vi "REF_EDITOR_prepare_DELETE_transaction.vi"(7 "nmb_of_top_rows (all)":i32, 8 "error_in":errorcluster, 10 "selected_record":i32, 11 "REF_EDIT_records":string[][](array[string])) -> (0 "error_out":errorcluster, 3 "DELETE_transaction":string[](array[string]))   [LabVIEW 2019]
uses:
  FGV/REF_EDITOR_records_display/FGV_REF_EDITOR_records_display.ctl
  FGV/login/FGV_login.ctl
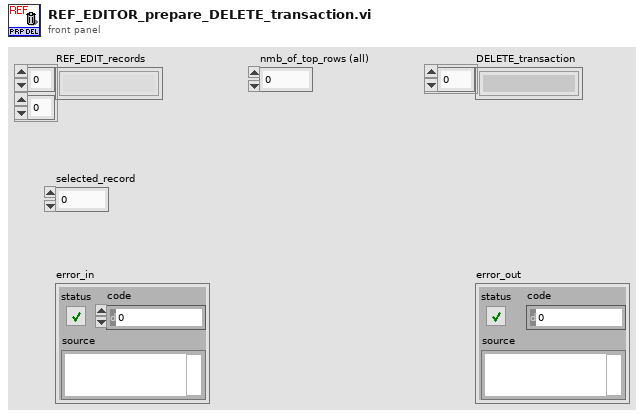
[diagram p1: front panel]
types:
  T1 = typedef "FGV_login.ctl" = enum16{"initialize", "login", "logout", "get_login_info"}
  T2 = typedef "FGV_REF_EDITOR_records_display.ctl" = enum16{"initialize", "set_reference_tables_names", "set_station_number", "set_type_filter", "set_headers", "set_records", "get_ref_table_name", "get_ref_hist_table_name", "get_station_number", "get_type_filter", "get_headers", "get_uneditable_columns", "get_all_info", "record_added?", "record_inserted?", "record_edited?", "record_updated?", "record_deleted?", "discard_changes"}
  T3 = typedef "REF_EDITOR_all_info.ctl" = cluster{"station_number":string, "type_filter":string, "reference_table":string, "reference_history":string, "headers":string[], "uneditable_columns":string[], "uneditable_columns":i32[], "editable_columns":i32[], "values_in_database":string[][], "size":cluster{"columns":i32, "SQL_rows":i32, "disp_rows":i32}, "REF_record_states":T4[]}
  T4 = typedef "SQL_record_states.ctl" = enum16{"Equal", "Added", "Edited", "Deleted"}
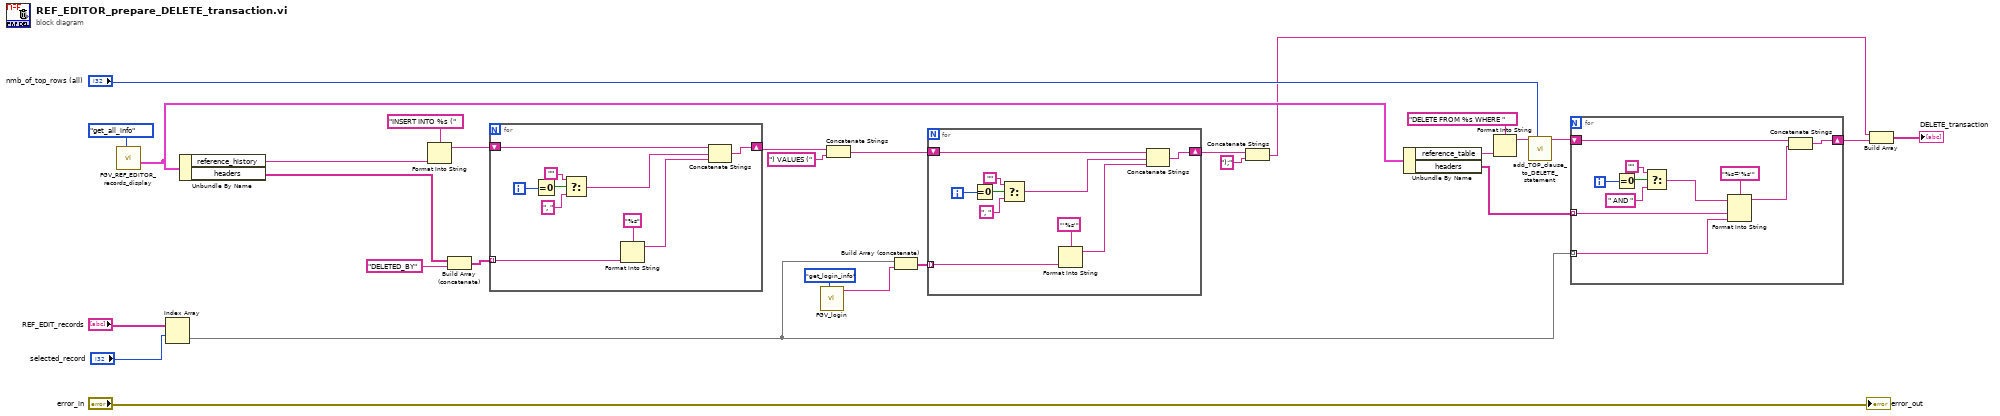
[diagram p0: block diagram]
diagram:
  n1 = call "FGV_REF_EDITOR_records_display.vi"("options"=FGV_REF_EDITOR_records_display."get_all_info") -> ("all_info"=w12:T3)  [unwired: 7 in, 3 out]
  n2 = Index Array(array="REF_EDIT_records", index (row)="selected_record") -> (element=w1:string[])  [unwired: 1 in]
  n3 = Unbundle By Name(w12) -> ("reference_history"=w11:string, "headers"=w9:string[])
  n4 = Format Into String(format string="INSERT INTO %s (", w11) -> (resulting string=w18:string)  [unwired: 2 in, 1 out]
  n5 = Build Array (concatenate)(w9, "DELETED_BY" ("reference_history")) -> (w8:string[])
  n6 = for {
    tunnel: w8 -> [w32] mode=indexing
    shift-right: [w34] -> w20
    shift-left: w18 -> [w35]
    i -> [w39]
    n7 = Equal To 0?(x=w39) -> (x = 0?=w38:bool)
    n8 = Select(t="", s=w38, f=", ") -> (s? t:f=w33:string)
    n9 = Format Into String(format string="%s", w32) -> (resulting string=w31:string)  [unwired: 2 in, 1 out]
    n10 = Concatenate Strings(w35, w33, w31) -> (w34:string)
  }
  n11 = call "FGV_login.vi"("options"=FGV_login."get_login_info") -> ("username_out"=w4:string)  [unwired: 8 in, 2 out]
  n12 = Concatenate Strings(w20, ") VALUES (" ("string")) -> (w15:string)
  n13 = Build Array (concatenate)(w1, w4) -> (w6:string[])
  n14 = for {
    tunnel: w6 -> [w42] mode=indexing
    shift-right: [w44] -> w13
    shift-left: w15 -> [w45]
    i -> [w49]
    n15 = Equal To 0?(x=w49) -> (x = 0?=w48:bool)
    n16 = Select(t="", s=w48, f=", ") -> (s? t:f=w43:string)
    n17 = Format Into String(format string="'%s'", w42) -> (resulting string=w41:string)  [unwired: 2 in, 1 out]
    n18 = Concatenate Strings(w45, w43, w41) -> (w44:string)
  }
  n19 = Concatenate Strings(w13, ");" ("string")) -> (w10:string)
  n20 = Unbundle By Name(w12) -> ("reference_table"=w24:string, "headers"=w25:string[])
  n21 = Format Into String(format string="DELETE FROM %s WHERE ", w24) -> (resulting string=w27:string)  [unwired: 2 in, 1 out]
  n22 = call "add_TOP_clause_to_DELETE_statement.vi"("nmb_of_top_rows (all)"="nmb_of_top_rows (all)", "DELETE_statement_in"=w27) -> ("DELETE_statement_out"=w29:string)  [unwired: 8 in, 1 out]
  n23 = for {
    tunnel: w1 -> [w52] mode=indexing
    tunnel: w25 -> [w53] mode=indexing
    shift-right: [w50] -> w22
    shift-left: w29 -> [w56]
    i -> [w60]
    n24 = Equal To 0?(x=w60) -> (x = 0?=w59:bool)
    n25 = Select(t="", s=w59, f=" AND ") -> (s? t:f=w54:string)
    n26 = Format Into String(format string="%s='%s'", initial string=w54, w53, w52) -> (resulting string=w51:string)  [unwired: 1 in, 1 out]
    n27 = Concatenate Strings(w56, w51) -> (w50:string)
  }
  n28 = Build Array(w10, w22) -> (→"DELETE_transaction":string[])
  "error_out" <- "error_in"
